vi "Timestamp Conversion.vi"   [LabVIEW 2026, in "synnax_clib.lvlib"]
uses:
  synnax_clib.lvlib
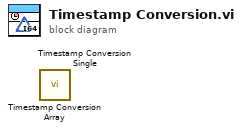
[diagram p0: block diagram]
diagram:
  n1 = call "Timestamp Conversion Array.vi"() -> ()  [unwired: 10 in, 1 out]
  n2 = call "Timestamp Conversion Single.vi"() -> ()  [unwired: 10 in, 1 out]
